vi "rt_loop_data_file_transmission.vi"(8 "error in (no error)":errorcluster caption="错误输入（无错误）", 10 "FTP Connection Parameters":T1={"host IP"="192.168.16.202", "port (21)"=21, "user"="Arthur", "password"="Alin@iHome301", "remote base path"="baofu\\"} caption="FTP连接参数", 11 "Message Queues":T2 caption="消息队列") -> (0 "error out":errorcluster caption="错误输出")   [LabVIEW 2015]
uses:
  support_vis/message_queue/all_rt_message_queues.ctl
  support_vis/message_queue/message_cluster.ctl
  globals/global_all_rt_loop_stop.vi
  <vilib>/FTP/NI_FTP.lvlib
  support_vis/message_queue/message_queue.lvlib
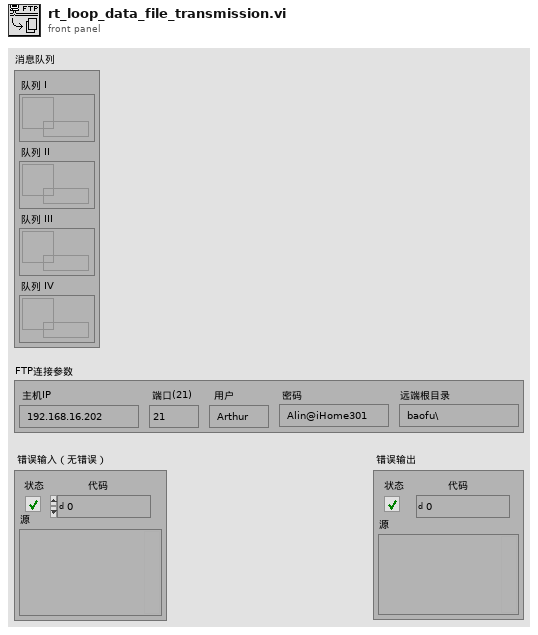
[diagram p1: front panel]
types:
  T1 = cluster{"host IP":string, "port (21)":u16, "user":string, "password":string, "remote base path":string}
  T2 = typedef "message_queue.lvlib/all_rt_message_queues.ctl" = cluster{"Queue I":refnum<queue>, "Queue II":refnum<queue>, "Queue III":refnum<queue>, "Queue IV":refnum<queue>}
  T3 = cluster{"remote path":string, "local path":path, "binary":bool, "data":string}
  T4 = typedef "NI_FTP.lvlib/FTP Session.ctl" = refnum<k5>
  T5 = cluster{"remote path":string, "local path":path, "binary":bool, "data":string}[]
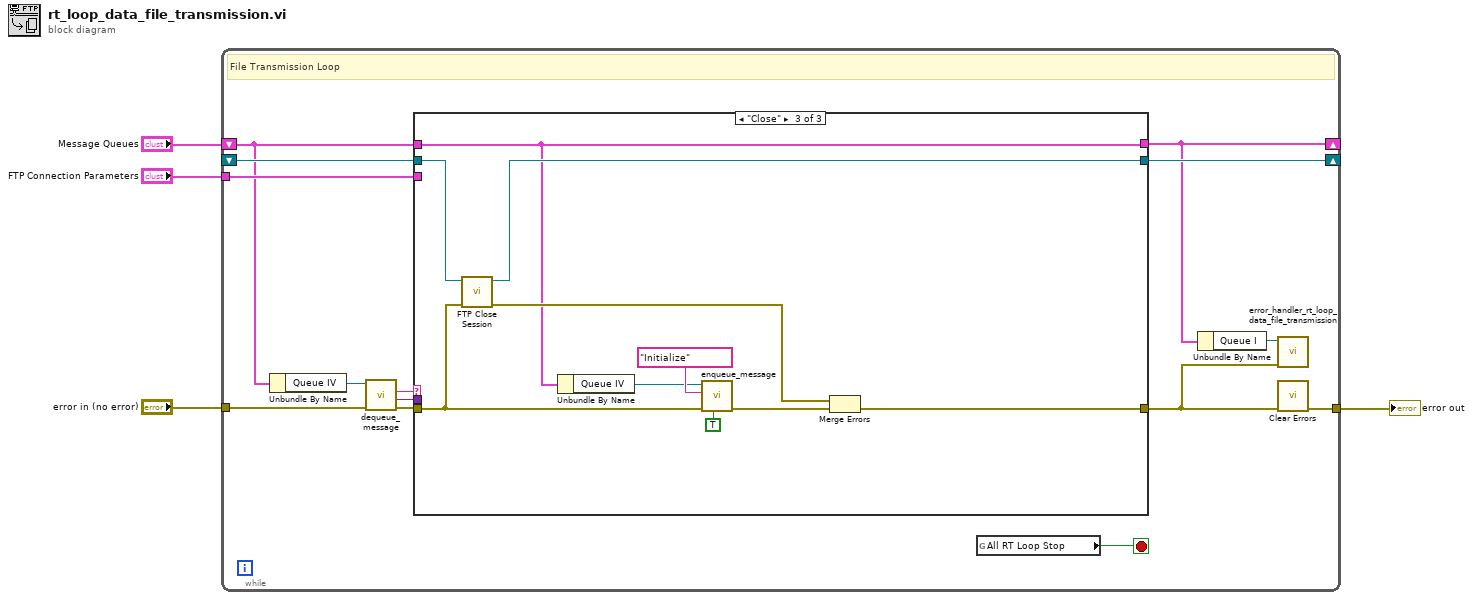
[diagram p0: block diagram]
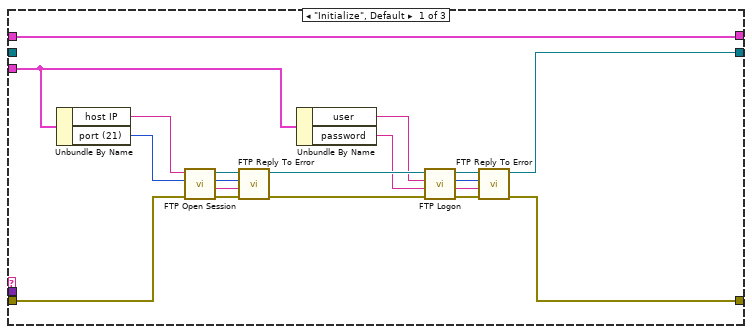
[diagram p2: hidden frame]
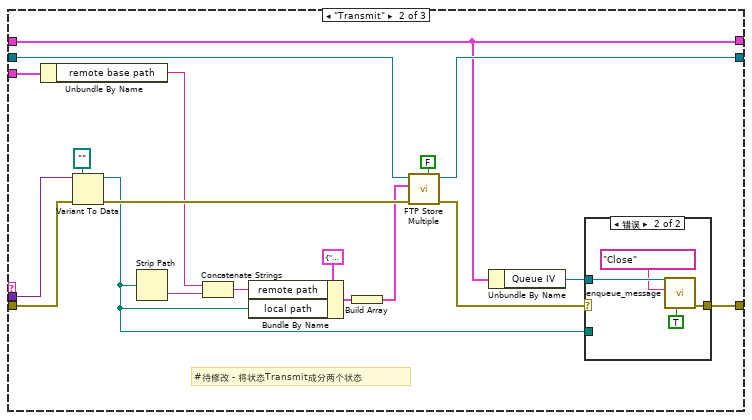
[diagram p3: hidden frame]
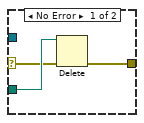
[diagram p4: hidden frame]
diagram:
  n1 = while {
    tunnel: "error in (no error)" -> [w15]
    tunnel: [w7] -> w4
    shift-right: [w16] -> _
    shift-left: _ -> [w18]
    shift-right: [w10] -> _
    shift-left: "Message Queues" -> [w5]
    tunnel: "FTP Connection Parameters" -> [w6]
    stop <- w17 stop-if-true
    # "File Transmission Loop"
    n2 = Unbundle By Name(w5) -> ("Queue IV"=w11:refnum<queue>)
    n3 = call "dequeue_message.vi"("error in (no error)"=w15, "Message Queue"=w11) -> ("error out"=w14:errorcluster, "Message Data"=w12:variant, "Message"=w13:string)  [unwired: 6 in, 1 out]
    n4 = case shown="\"Close\"" w13 {
      tunnel: w12 -> [_ w50 _]
      tunnel: w18 -> [_ w56 w73]
      tunnel: [w25 w52 w67] -> w8
      tunnel: w14 -> [w26 w53 w65]
      tunnel: [w27 w55 w72] -> w16
      tunnel: [w24 w43 w64] -> w10
      tunnel: w5 -> [w24 w43 w64]
      tunnel: w6 -> [w19 w40 _]
      frame "Initialize", Default {
        n5 = Unbundle By Name(w19) -> ("host IP"=w22:string, "port (21)"=w23:u16)
        n6 = call <vilib>:"FTP Open Session.vi"("error in (no error)"=w26, "remote port (21)"=w23, "address"=w22) -> ("error out"=w28:errorcluster, "reply string"=w31:string, "reply code"=w30:i32, "ftp session"=w29:T4)  [unwired: 1 in, 4 out]
        n7 = call <vilib>:"FTP Reply To Error.vi"("error in (no error)"=w28, "reply string in"=w31, "reply code in"=w30, "ftp session"=w29) -> ("error out"=w33:errorcluster, "ftp session out"=w32:T4)  [unwired: 2 out]
        n8 = Unbundle By Name(w19) -> ("user"=w20:string, "password"=w21:string)
        n9 = call <vilib>:"FTP Logon.vi"("error in (no error)"=w33, "password"=w21, "user"=w20, "ftp session"=w32) -> ("error out"=w34:errorcluster, "reply string"=w37:string, "reply code"=w36:i32, "ftp session out"=w35:T4)  [unwired: 4 out]
        n10 = call <vilib>:"FTP Reply To Error.vi"("error in (no error)"=w34, "reply string in"=w37, "reply code in"=w36, "ftp session"=w35) -> ("error out"=w25:errorcluster, "ftp session out"=w27:T4)  [unwired: 2 out]
      }
      frame "Transmit" {
        # "#待修改 - 将状态Transmit成分两个状态"
        n11 = Unbundle By Name(w40) -> ("remote base path"=w39:string)
        n12 = Variant To Data(error in=w53, type=path "", Variant=w50) -> (data=w44:path, error out=w51:errorcluster)
        n13 = Strip Path(path=w44) -> (name=w41:string)  [unwired: 1 out]
        n14 = Concatenate Strings(w39, w41) -> (w38:string)
        n15 = Bundle By Name(cluster=T3 {"remote path"="", "local path"=path "", "binary"=TRUE, "data"=""} ("transfer spec"), "remote path"=w38, "local path"=w44) -> (w46:T3)
        n16 = Build Array(w46) -> (w45:T5)
        n17 = call <vilib>:"FTP Store Multiple.vi"("active (T)"=FALSE, "error in (no error)"=w51, "file specifications"=w45, "ftp session"=w56) -> ("error out"=w54:errorcluster, "ftp session out"=w55:T4)  [unwired: 6 out]
        n18 = Unbundle By Name(w43) -> ("Queue IV"=w42:refnum<queue>)
        n19 = case shown="错误" w54 {
          selector: w54 -> [w58 _]
          tunnel: [w57 w63] -> w52
          tunnel: w44 -> [w59 _]
          tunnel: w42 -> [_ w62]
          frame No Error {
            n20 = Delete(path (use dialog)=w59, error in=w58) -> (error out=w57:errorcluster)  [unwired: 3 in, 2 out]
          }
          frame Error {
            n21 = call "enqueue_message.vi"("Priority Message? (F)"=TRUE, "Message"="Close", "Message Queue"=w62) -> ("error out"=w63:errorcluster)  [unwired: 7 in, 1 out]
          }
        }
      }
      frame "Close" {
        n22 = call <vilib>:"FTP Close Session.vi"("error in (no error)"=w65, "ftp session"=w73) -> ("error out"=w66:errorcluster, "ftp session out"=w72:T4)  [unwired: 6 in, 2 out]
        n23 = Unbundle By Name(w64) -> ("Queue IV"=w69:refnum<queue>)
        n24 = call "enqueue_message.vi"("Priority Message? (F)"=TRUE, "error in (no error)"=w65, "Message"="Initialize", "Message Queue"=w69) -> ("error out"=w71:errorcluster)  [unwired: 6 in, 1 out]
        n25 = Merge Errors(w66, w71) -> (w67:errorcluster)
      }
    }
    n26 = global read "global_all_rt_loop_stop.vi" "All RT Loop Stop"() -> (w17:bool)
    n27 = Unbundle By Name(w10) -> ("Queue I"=w9:refnum<queue>)
    n28 = call "error_handler_rt_loop_data_file_transmission.vi"("error in (no error)"=w8, "Message Queue"=w9) -> ()  [unwired: 9 in, 1 out]
    n29 = call <vilib>:"Clear Errors.vi"("error in (no error)"=w8) -> ("error out"=w7:errorcluster)  [unwired: 5 in, 1 out]
  }
  "error out" <- w4
